vi "RecordingControl_SetFileName.vi"(8 "error in (no error)":errorcluster, 10 "File Name or Path":path, 11 "OXY_SCPI Reseource In":refnum<visa-resource-name>) -> (0 "error out":errorcluster, 1 "communication_data":T1, 3 "OXY_SCPI Reseource Out":refnum<visa-resource-name>)   [LabVIEW 2018, in "OXYGEN.lvlib"]
doc: "Set File Name or Path of the Recording File."
uses:
  OXYGEN.lvlib
  TypeDefs/Cluster_RawCommData.ctl
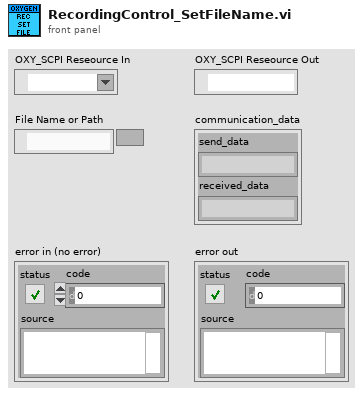
[diagram p1: front panel]
types:
  T1 = typedef "OXYGEN.lvlib/Cluster_RawCommData.ctl" = cluster{"send_data":string, "received_data":string}
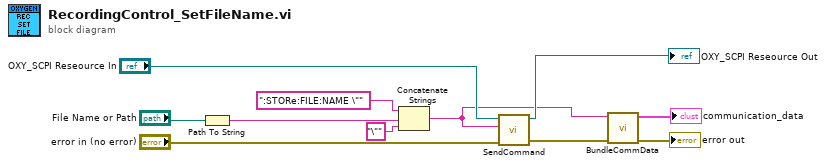
[diagram p0: block diagram]
diagram:
  n1 = Path To String(path="File Name or Path") -> (string=w5:string)
  n2 = Concatenate Strings(":STORe:FILE:NAME \"", w5, "\"") -> (w3:string)
  n3 = call "SendCommand.vi"("error in (no error)"="error in (no error)", "String to Send"=w3, "OXY_SCPI Reseource In"="OXY_SCPI Reseource In") -> ("error out"=w4:errorcluster, "OXY_SCPI Reseource Out"=→"OXY_SCPI Reseource Out":refnum<visa-resource-name>)  [unwired: 7 in]
  n4 = call "BundleCommData.vi"("error in (no error)"=w4, "send_data"=w3) -> ("error out"=→"error out":errorcluster, "communication_data"=→"communication_data":T1)  [unwired: 8 in]
